vi "PWM Configure Port.vi"(0 "Arduino Resource":T1={"VISA resource"="", "Board Type"=enum."Uno", "Connection Type"=enum."USB / Serial", "Bytes Per Packet (15)"=15}, 5 "PWM Pin (3)":u8, 7 "PWM Pin (5)":u8, 9 "PWM Pin (6)":u8, 11 "error in":errorcluster) -> (4 "Arduino Resource":T1={"VISA resource"="", "Board Type"=enum."Uno", "Connection Type"=enum."USB / Serial", "Bytes Per Packet (15)"=15}, 8 "PWM Pins":u8[](array[numeric]), 15 "error out":errorcluster)   [LabVIEW 2015, in "LabVIEW Interface for Arduino.lvlib"]
doc: "Configure 3 Arduino pins to use for PWM."
uses:
  <vilib>/LabVIEW Interface for Arduino/LabVIEW Interface for Arduino.lvlib
  <vilib>/LabVIEW Interface for Arduino/Type Defs/Arduino Resource.ctl
  <vilib>/LabVIEW Interface for Arduino/Type Defs/Board Type.ctl
  <vilib>/LabVIEW Interface for Arduino/Type Defs/Pin Mode.ctl
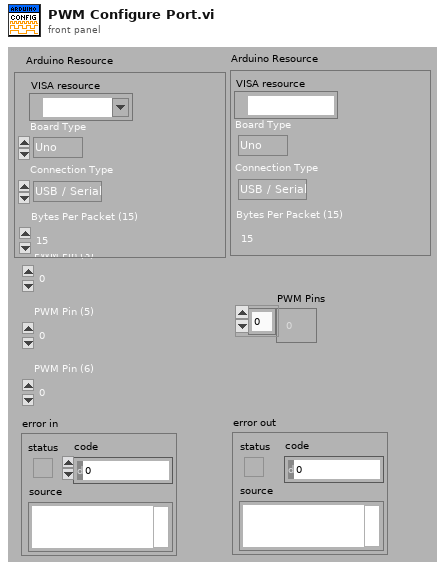
[diagram p1: front panel]
types:
  T1 = typedef "LabVIEW Interface for Arduino.lvlib/Arduino Resource.ctl" = cluster{"VISA resource":refnum<visa-resource-name>, "Board Type":T2, "Connection Type":enum8{"USB / Serial"}, "Bytes Per Packet (15)":u8}
  T2 = typedef "LabVIEW Interface for Arduino.lvlib/Board Type.ctl" = enum16{"Uno", "Dimuelanove w/Atmega 328", "Mega 2560"}
  T3 = typedef "LabVIEW Interface for Arduino.lvlib/Pin Mode.ctl" = enum8{"Input", "Output"}
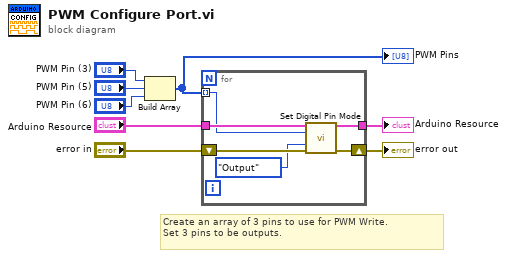
[diagram p0: block diagram]
diagram:
  # "Create an array of 3 pins to use for PWM Write.\nSet 3 pins to be outputs."
  n1 = Build Array("PWM Pin (3)", "PWM Pin (5)", "PWM Pin (6)") -> (w1:u8[])
  "PWM Pins" <- w1
  n2 = for {
    tunnel: "Arduino Resource" -> [w14]
    tunnel: [w13] -> w4
    tunnel: w1 -> [w10] mode=indexing
    shift-right: [w11] -> w2
    shift-left: "error in" -> [w12]
    n3 = call <vilib>:"Set Digital Pin Mode.vi"("Arduino Resource"=w14, "Digital I/O Pin"=w10, "Pin Mode (Input)"=Pin_Mode."Output" ("Pin Mode"), "error in"=w12) -> ("Arduino Resource"=w13:T1, "error out"=w11:errorcluster)  [unwired: 10 in]
  }
  "error out" <- w2
  "Arduino Resource" <- w4
